vi "(SubVI)_2DPSF_CreateFile_v17.vi"(9 "Imp tab Label":string, 10 "Imp Tab Parameters":T1, 11 "Path":path=path "C:/OCT_Data") -> (0 "error out":errorcluster, 3 "Doppler_Data_File":refnum<file>)   [LabVIEW 2019]
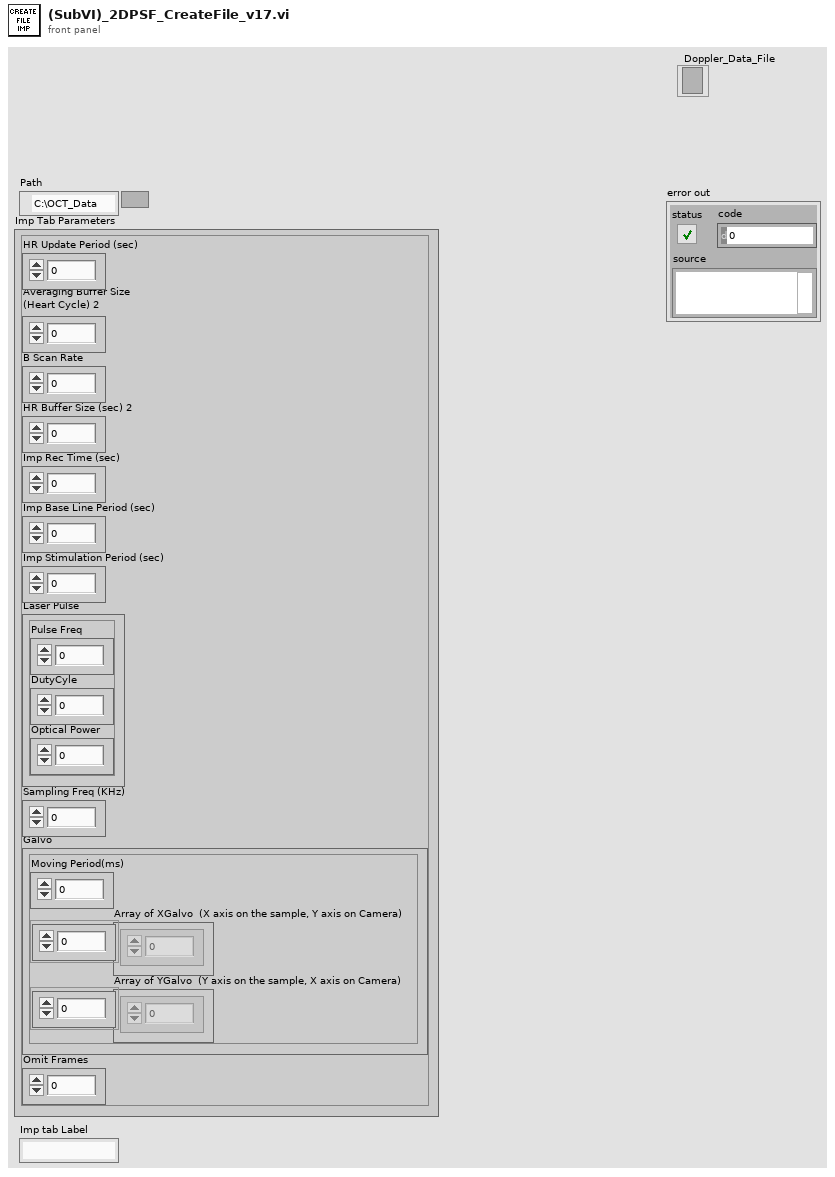
[diagram p1: front panel]
types:
  T1 = cluster{"HR Update Period (sec)":i32, "Averaging Buffer Size\n(Heart Cycle) 2":dbl, "B Scan Rate":dbl, "HR Buffer Size (sec) 2":dbl, "Imp Rec Time (sec)":dbl, "Imp Base Line Period (sec)":dbl, "Imp Stimulation Period (sec)":dbl, "Laser Pulse":cluster{"Pulse Freq":dbl, "DutyCyle":dbl, "Optical Power":dbl}, "Sampling Freq (KHz)":dbl, "Galvo":cluster{"Moving Period(ms)":dbl, "Array of XGalvo  (X axis on the sample, Y axis on Camera)":dbl[], "Array of YGalvo  (Y axis on the sample, X axis on Camera)":dbl[]}, "Omit Frames":i32}
  T2 = enum16{"big-endian, network order", "native, host order", "little-endian"}
  T3 = enum16{"open", "replace", "create", "open or create", "replace or create", "replace or create with confirmation"}
  T4 = cluster{"Pulse Freq":dbl, "DutyCyle":dbl, "Optical Power":dbl}
  T5 = cluster{"Moving Period(ms)":dbl, "Array of XGalvo  (X axis on the sample, Y axis on Camera)":dbl[], "Array of YGalvo  (Y axis on the sample, X axis on Camera)":dbl[]}
  T6 = cluster{"string":string, dbl, "string":string, "Averaging Buffer Size\n(Heart Cycle) 2":dbl, "string":string, "B Scan Rate":dbl, "string":string, "HR Buffer Size (sec) 2":dbl}
  T7 = cluster{"string":string, "Imp Rec Time (sec)":dbl, "string":string, "Imp Base Line Period (sec)":dbl, "string":string, "Imp Stimulation Period (sec)":dbl}
  T8 = cluster{"string":string, "Pulse Freq":dbl, "string":string, "DutyCyle":dbl, "string":string, "Optical Power":dbl}
  T9 = cluster{"string":string, "string":string, "string":string, "Scan Angle 2D":dbl}
  T10 = cluster{"string":string, "Sampling Freq (KHz)":dbl, "string":string, "Moving Period(ms)":dbl, "string":string, dbl, "string":string, "Array of XGalvo  (X axis on the sample, Y axis on Camera)":dbl[], "string":string, dbl, "string":string, "Array of YGalvo  (Y axis on the sample, X axis on Camera)":dbl[], "string":string, dbl}
  T11 = cluster{cluster{"string":string, "string":string, "string":string, "Scan Angle 2D":dbl}, cluster{"string":string, dbl, "string":string, "Averaging Buffer Size\n(Heart Cycle) 2":dbl, "string":string, "B Scan Rate":dbl, "string":string, "HR Buffer Size (sec) 2":dbl}, cluster{"string":string, "Imp Rec Time (sec)":dbl, "string":string, "Imp Base Line Period (sec)":dbl, "string":string, "Imp Stimulation Period (sec)":dbl}, cluster{"string":string, "Pulse Freq":dbl, "string":string, "DutyCyle":dbl, "string":string, "Optical Power":dbl}, cluster{"string":string, "Sampling Freq (KHz)":dbl, "string":string, "Moving Period(ms)":dbl, "string":string, dbl, "string":string, "Array of XGalvo  (X axis on the sample, Y axis on Camera)":dbl[], "string":string, dbl, "string":string, "Array of YGalvo  (Y axis on the sample, X axis on Camera)":dbl[], "string":string, dbl}, "string":string, "string":string}
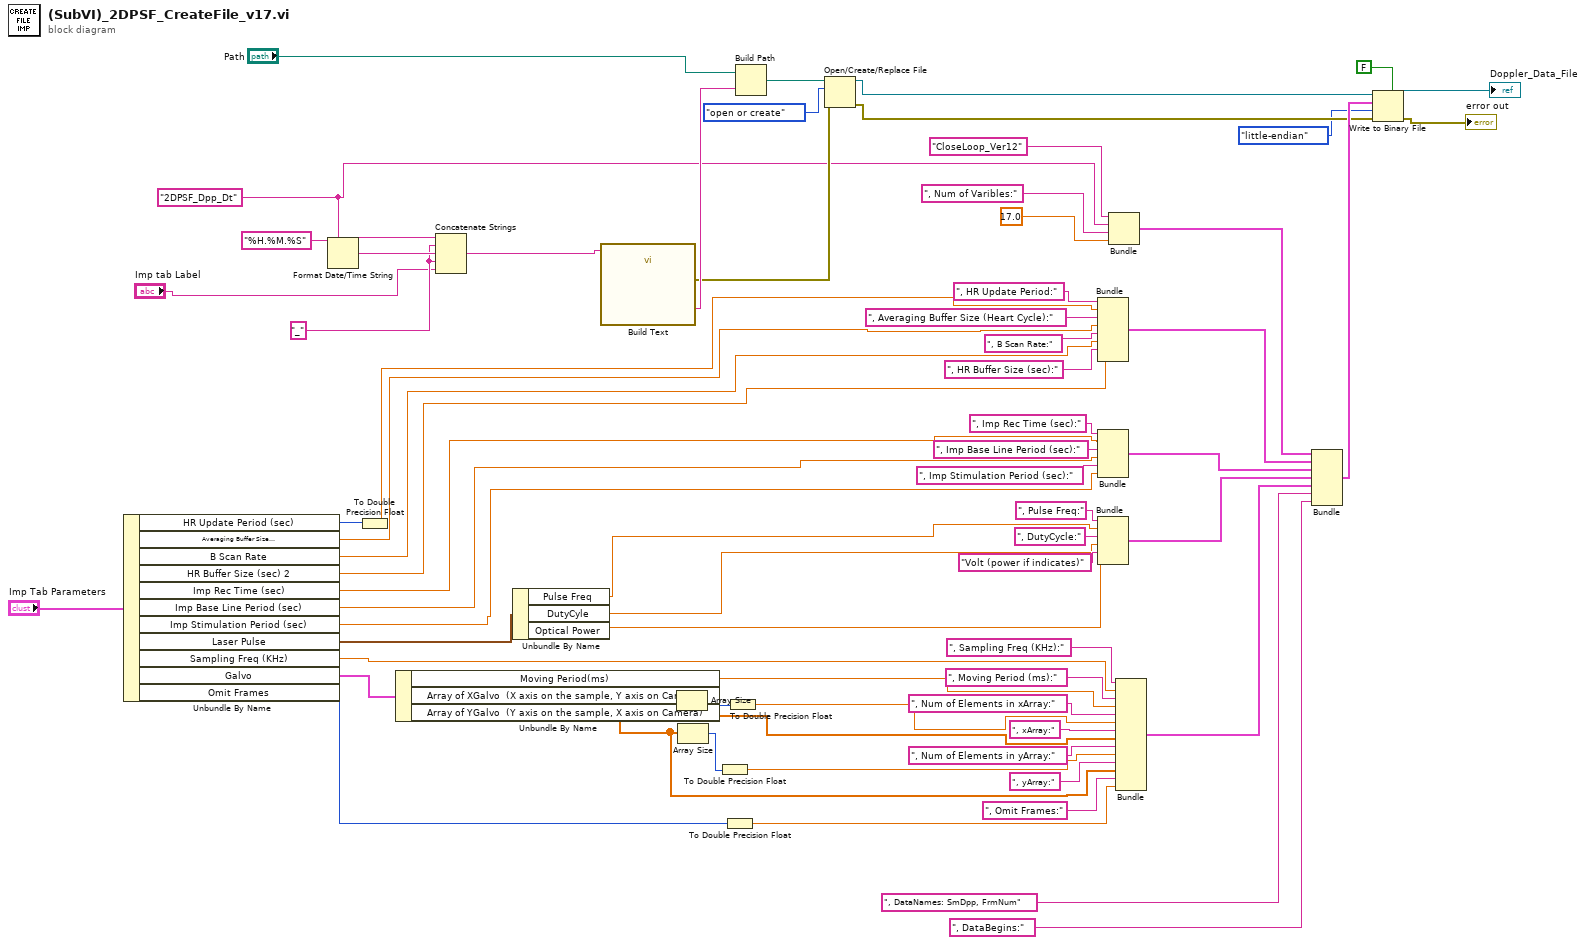
[diagram p0: block diagram]
diagram:
  w31 = "2DPSF_Dpp_Dt" ("string")
  w65 = "_" ("3D Label")
  n1 = Unbundle By Name("Imp Tab Parameters") -> ("HR Update Period (sec)"=w29:i32, "Averaging Buffer Size\n(Heart Cycle) 2"=w28:dbl, "B Scan Rate"=w26:dbl, "HR Buffer Size (sec) 2"=w24:dbl, "Imp Rec Time (sec)"=w23:dbl, "Imp Base Line Period (sec)"=w21:dbl, "Imp Stimulation Period (sec)"=w20:dbl, "Laser Pulse"=w19:T4, "Sampling Freq (KHz)"=w11:dbl, "Galvo"=w14:T5, "Omit Frames"=w3:i32)
  n2 = Format Date/Time String(time format string (%c)="%H.%M.%S") -> (date/time string=w68:string)  [unwired: 2 in]
  n3 = To Double Precision Float(number=w29) -> (double precision float=w18:dbl)
  n4 = Unbundle By Name(w14) -> ("Moving Period(ms)"=w13:dbl, "Array of XGalvo  (X axis on the sample, Y axis on Camera)"=w9:dbl[], "Array of YGalvo  (Y axis on the sample, X axis on Camera)"=w7:dbl[])
  n5 = Concatenate Strings(w31, w65, w68, w65, "Imp tab Label") -> (w67:string)
  n6 = Unbundle By Name(w19) -> ("Pulse Freq"=w17:dbl, "DutyCyle"=w16:dbl, "Optical Power"=w15:dbl)
  n7 = call "Build Text"("Beginning Text"=w67) -> ("Result"=w66:string, "error out"=w35:errorcluster)  [unwired: 13 in]
  n8 = Array Size(array=w9) -> (size(s)=w10:i32)
  n9 = Array Size(array=w7) -> (size(s)=w8:i32)
  n10 = To Double Precision Float(number=w8) -> (double precision float=w5:dbl)
  n11 = To Double Precision Float(number=w3) -> (double precision float=w2:dbl)
  n12 = To Double Precision Float(number=w10) -> (double precision float=w6:dbl)
  n13 = Build Path(base path="Path", name or relative path=w66) -> (appended path=w64:path)
  n14 = Open/Create/Replace File(file path (use dialog)=w64, error in=w35, operation (0:open)=T3."open or create") -> (refnum out=w60:refnum<file>, error out=w59:errorcluster)  [unwired: 3 in, 1 out]
  n15 = Bundle("string"=", HR Update Period:", w18, "string"=", Averaging Buffer Size (Heart Cycle):", "Averaging Buffer Size\n(Heart Cycle) 2"=w28, "string"=", B Scan Rate:", "B Scan Rate"=w26, "string"=", HR Buffer Size (sec):", "HR Buffer Size (sec) 2"=w24) -> (w40:T6)  [unwired: 1 in]
  n16 = Bundle("string"=", Imp Rec Time (sec):", "Imp Rec Time (sec)"=w23, "string"=", Imp Base Line Period (sec):", "Imp Base Line Period (sec)"=w21, "string"=", Imp Stimulation Period (sec):", "Imp Stimulation Period (sec)"=w20) -> (w39:T7)  [unwired: 1 in]
  n17 = Bundle("string"=", Pulse Freq:", "Pulse Freq"=w17, "string"=", DutyCycle:", "DutyCyle"=w16, "string"="Volt (power if indicates)", "Optical Power"=w15) -> (w38:T8)  [unwired: 1 in]
  n18 = Bundle("string"="CloseLoop_Ver12", "string"=w31, "string"=", Num of Varibles:", "Scan Angle 2D"=17.0) -> (w62:T9)  [unwired: 1 in]
  n19 = Bundle("string"=", Sampling Freq (KHz):", "Sampling Freq (KHz)"=w11, "string"=", Moving Period (ms):", "Moving Period(ms)"=w13, "string"=", Num of Elements in xArray:", w6, "string"=", xArray:", "Array of XGalvo  (X axis on the sample, Y axis on Camera)"=w9, "string"=", Num of Elements in yArray:", w5, "string"=", yArray:", "Array of YGalvo  (Y axis on the sample, X axis on Camera)"=w7, "string"=", Omit Frames:", w2) -> (w37:T10)  [unwired: 1 in]
  n20 = Bundle(w62, w40, w39, w38, w37, "string"=", DataNames: SmDpp, FrmNum", "string"=", DataBegins:") -> (w61:T11)  [unwired: 1 in]
  n21 = Write to Binary File(file (use dialog)=w60, data=w61, error in=w59, 5:FALSE ("prepend array or string size? (T)"), 9:T2."little-endian" ("byte order (0:big-endian, network order)")) -> (refnum out=→"Doppler_Data_File":refnum<file>, error out=→"error out":errorcluster)  [unwired: 1 in, 1 out]
